vi "PFI-28000-Channel_Get Test Mode.vi"(8 "error in (no error)":errorcluster, 11 "PFI-28000-Channel in":refnum<class "PFI-28000-Channel.lvclass">) -> (0 "error out":errorcluster, 2 "Test Mode":string, 3 "PFI-28000-Channel out":refnum<class "PFI-28000-Channel.lvclass">)   [LabVIEW 2017, in "PFI-28000-Channel.lvclass"]
uses:
  PFI-28000-Channel.lvclass
  Utilities/PFI-28000-Utils.lvlib
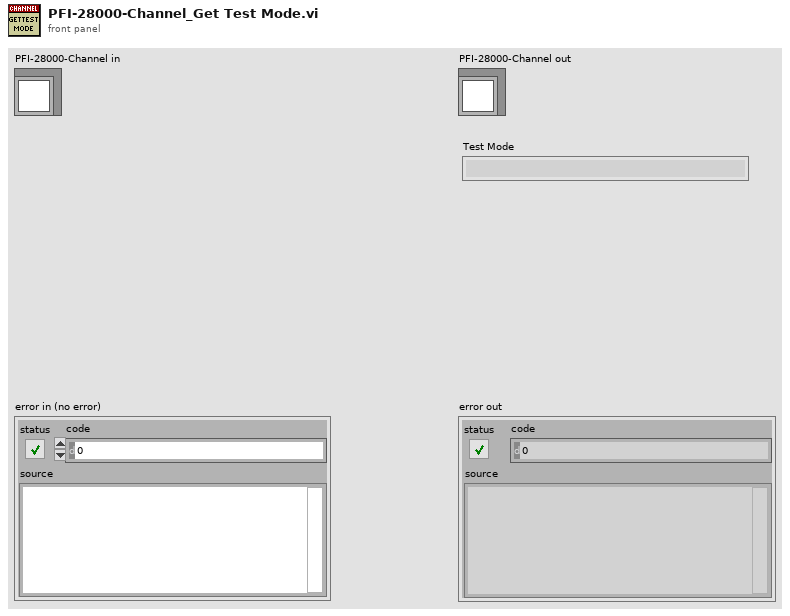
[diagram p1: front panel]
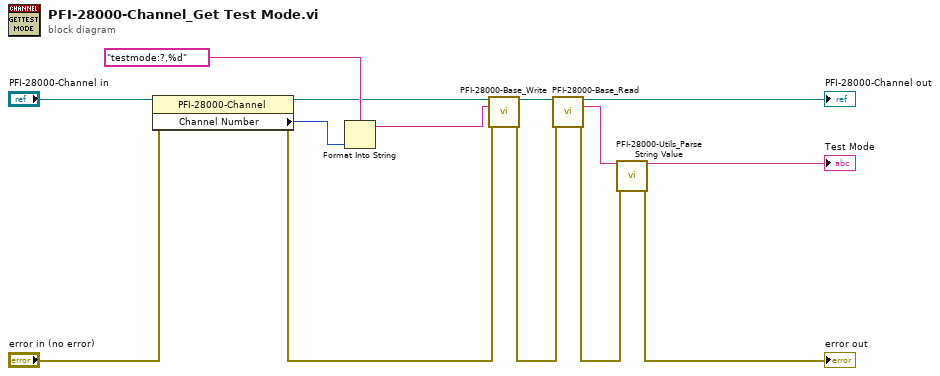
[diagram p0: block diagram]
diagram:
  n1 = property class="PFI-28000-Channel"(reference="PFI-28000-Channel in", error in="error in (no error)") -> (reference out=w5:refnum<class "PFI-28000-Channel.lvclass">, error out=w8:errorcluster, "Channel Number"=w10:i32)
  n2 = Format Into String(format string="testmode:?,%d" ("empty string"), w10) -> (resulting string=w7:string)  [unwired: 2 in, 1 out]
  n3 = call-dynamic "PFI-28000-Base_Write.vi"("PFI-28000-Base in"=w5, "Command"=w7, "error in (no error)"=w8) -> ("PFI-28000-Base out"=w14:refnum<class "PFI-28000-Channel.lvclass">, "error out"=w12:errorcluster)  [unwired: 11 in]
  n4 = call-dynamic "PFI-28000-Base_Read.vi"("PFI-28000-Base in"=w14, "error in (no error)"=w12) -> ("PFI-28000-Base out"=→"PFI-28000-Channel out":refnum<class "PFI-28000-Channel.lvclass">, "Response"=w4:string, "error out"=w2:errorcluster)  [unwired: 10 in, 1 out]
  n5 = call "PFI-28000-Utils_Parse String Value.vi"("String"=w4, "error in (no error)"=w2) -> ("String Value"=→"Test Mode":string, "error out"=→"error out":errorcluster)  [unwired: 11 in, 1 out]
